vi "view ALR_1.vi"(6 "ALRNames":refnum<data-value>, 9 "ALR_ON_OFF":refnum<data-value>, 10 "State":T1(array[cluster]), 11 "ActivateALRHandling":bool) -> (3 "This VI":refnum<vi>)   [LabVIEW 2019, in "Alarms.lvlib"]
uses:
  Alarms.lvlib
  Trigers/D^.vi
  Logik/fronts.vi
  Timer Delay/Timer.vi
  Counter/Counter.lvlib
panel:
  in  "n_elem":i32(c297)
  out "alrcode":string[](array[string])
  out "alr2":bool
  out "alr1":bool
  out "n alr":i32
  in  "block":bool[](array[boolean])=[FALSE, FALSE, FALSE, FALSE, FALSE, FALSE, FALSE, FALSE, FALSE, FALSE]
  in  "check":bool[](array[boolean])=[FALSE, FALSE, FALSE, FALSE, FALSE, FALSE, FALSE, FALSE, FALSE, FALSE]
  out "alrname":string[](array[string])
  out "t ms view":u32[](array[numeric])
  out "alr view":bool[](array[boolean])
  out "alr not block_view":bool[](array[boolean])
  out "alr on_view":bool[](array[boolean])
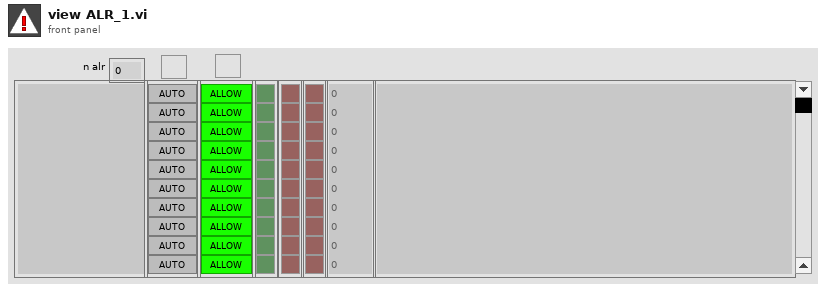
[diagram p1: front panel]
types:
  T1 = cluster{"ALR":bool, "ALR NOT block":bool, "ALR ON":bool, "t ms":u32, "alrnum":i32, "ack state":enum32{"not", "tripped", "reset", "ack"}, "color":u32, "alrname":string}[]
  T2 = enum32{"Invalid", "Standard", "Closed", "Hidden", "Minimized", "Maximized"}
  T3 = cluster{"ALR_ON":bool[], "ALR_OFF":bool[], "ALR_reset":bool[], "ALR_check":bool[], "ALR_block":bool[], "ALR_Ack":bool[]}
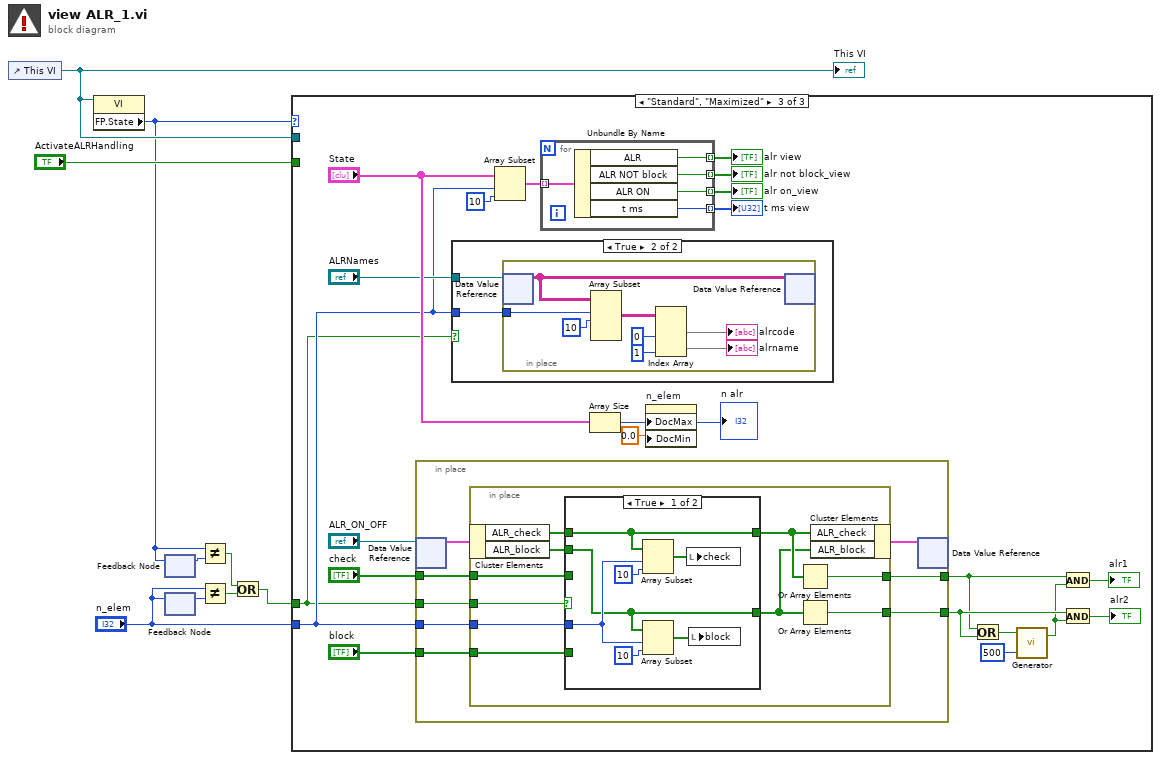
[diagram p0: block diagram]
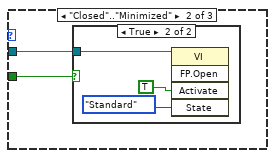
[diagram p3: hidden frame]
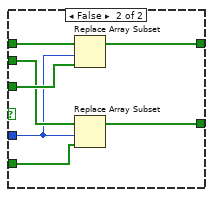
[diagram p5: hidden frame]
diagram:
  n1 = control-ref of="This VI"() -> (w7:refnum<vi>)
  "This VI" <- w7
  n2 = property class="VI"(reference=w7) -> ("FP.State"=w5:T2)  [unwired: 1 in, 2 out]
  n3 = feedback #1() -> (w6:T2)  [unwired: 1 in]
  n4 = feedback-in #1(w5) -> ()
  n5 = feedback #2() -> (w9:i32)  [unwired: 1 in]
  n6 = feedback-in #2("n_elem") -> ()
  n7 = Not Equal?(x=w5, y=w6) -> (x != y?=w4:bool)
  n8 = Not Equal?(x="n_elem", y=w9) -> (x != y?=w3:bool)
  n9 = Or(x=w4, y=w3) -> (x .or. y?=w2:bool)
  n10 = case shown="\"Standard\", \"Maximized\"" w5 {
    tunnel: "ActivateALRHandling" -> [_ w11 _]
    tunnel: w7 -> [_ w10 _]
    tunnel: w2 -> [_ _ w16]
    tunnel: "n_elem" -> [_ _ w17]
    frame "Invalid", Default {
    }
    frame "Closed".."Minimized" {
      n11 = case shown="True" w11 {
        tunnel: w10 -> [_ w12]
        frame False {
        }
        frame True {
          n12 = invoke class="VI" method="FP.Open"(reference=w12, "Activate"=TRUE ("Activate?"), "State"=T2."Standard") -> ()  [unwired: 2 in, 5 out]
        }
      }
    }
    frame "Standard", "Maximized" {
      n13 = in-place {
        in-place-border: w17 -> [w42]
        in-place-border: "check" -> [w41]
        in-place-border: "block" -> [w40]
        in-place-border: [w39] -> w25
        in-place-border: [w38] -> w26
        in-place-border: w16 -> [w37]
        n14 = in-place-dvr #3("ALR_ON_OFF") -> (w44:T3)  [unwired: 1 out]
        n15 = in-place {
          in-place-border: w42 -> [w50]
          in-place-border: w41 -> [w53]
          in-place-border: w40 -> [w51]
          in-place-border: [w47] -> w39
          in-place-border: [w46] -> w38
          in-place-border: w37 -> [w45]
          n16 = in-place-cluster #4(w44) -> ("ALR_check"=w54:bool[], "ALR_block"=w52:bool[])
          n17 = case shown="True" w45 {
            tunnel: w54 -> [w60 w67]
            tunnel: w53 -> [_ w68]
            tunnel: w52 -> [w55 w65]
            tunnel: w51 -> [_ w62]
            tunnel: w50 -> [w56 w63]
            tunnel: [w60 w66] -> w49
            tunnel: [w55 w64] -> w48
            frame True {
              n18 = Array Subset(array=w60, index=w56, length=10) -> (w59:bool[])
              n19 = Array Subset(array=w55, index=w56, length=10) -> (w57:bool[])
              n20 = local write "check"(w59) -> ()
              n21 = local write "block"(w57) -> ()
            }
            frame False {
              n22 = Replace Array Subset(array=w67, new element=w68, index=w63) -> (w66:bool[])
              n23 = Replace Array Subset(array=w65, new element=w62, index=w63) -> (w64:bool[])
            }
          }
          n24 = Or Array Elements(Boolean array=w49) -> (logical OR=w47:bool)
          n25 = Or Array Elements(Boolean array=w48) -> (logical OR=w46:bool)
          n26 = in-place-cluster #4("ALR_check"=w49, "ALR_block"=w48) -> (w43:T3)
        }
        n27 = in-place-dvr #3(w43) -> ()  [unwired: 2 out]
      }
      n28 = case shown="True" w16 {
        tunnel: w17 -> [_ w70]
        tunnel: "ALRNames" -> [_ w69]
        frame False {
        }
        frame True {
          n29 = in-place {
            in-place-border: w70 -> [w72]
            n30 = in-place-dvr #5(w69) -> (w71:string[][])  [unwired: 1 out]
            n31 = Array Subset(array=w71, index (row)=w72, length (row)=10 ("length")) -> (w73:string[][])  [unwired: 2 in]
            n32 = Index Array(array=w73, index (col) #1=0 ("index"), index (col) #2=1 ("index (col)")) -> (element #1=→"alrcode":string[], element #2=→"alrname":string[])  [unwired: 2 in]
            n33 = in-place-dvr #5(w71) -> ()  [unwired: 2 out]
          }
        }
      }
      n34 = Array Subset(array="State", index=w17, length=10) -> (w31:T1)
      n35 = for {
        tunnel: w31 -> [w83] mode=indexing
        tunnel: [w82] -> w36 mode=indexing
        tunnel: [w81] -> w35 mode=indexing
        tunnel: [w80] -> w34 mode=indexing
        tunnel: [w79] -> w33 mode=indexing
        n36 = Unbundle By Name(w83) -> ("ALR"=w82:bool, "ALR NOT block"=w81:bool, "ALR ON"=w80:bool, "t ms"=w79:u32)
      }
      "alr on_view" <- w34
      "alr not block_view" <- w35
      "alr view" <- w36
      "t ms view" <- w33
      n37 = Array Size(array="State") -> (size(s)=w30:i32)
      "n alr" <- w30
      n38 = property on="n_elem" class="Scroll (strict)"("DocMax"=w30, "DocMin"=0.0 ("Data Entry Limits:Minimum")) -> ()  [unwired: 2 in, 2 out]
      n39 = Or(x=w25, y=w26) -> (x .or. y?=w24:bool)
      n40 = call "Generator.vi"("T ms (500)"=u32 500 ("T (ms)"), "ON (F)"=w24) -> ("Q"=w22:bool)  [unwired: 2 in]
      n41 = And(x=w25, y=w22) -> (x .and. y?=→"alr1":bool)
      n42 = And(x=w26, y=w22) -> (x .and. y?=→"alr2":bool)
    }
  }
